vi "Read_Instr.vi"(8 "error in (no error)":errorcluster caption="entrée d'erreur (pas d'erreur)", 11 "Class Instrument Multimeter en entrée":refnum<class "Class Instrument LED_Analyser.lvclass">) -> (0 "error out":errorcluster caption="sortie d'erreur", 3 "Class Instrument Multimeter en sortie":refnum<class "Class Instrument LED_Analyser.lvclass">)   [LabVIEW 2020, in "Library Instrument & Equipement.lvlib" / "Library Instruments.lvlib" / "Class Instrument LED_Analyser.lvclass"]
uses:
  Class Instrument LED_Analyser.lvclass
  Class Instrument LED_Analyser.lvclass/Class Instrument LED_Analyser.ctl
  Instrument (Default)/Class Instrument (Default).lvclass
  LED Analyser/Class Led Analyser (Default)/Class LED Analyser (Default).lvclass
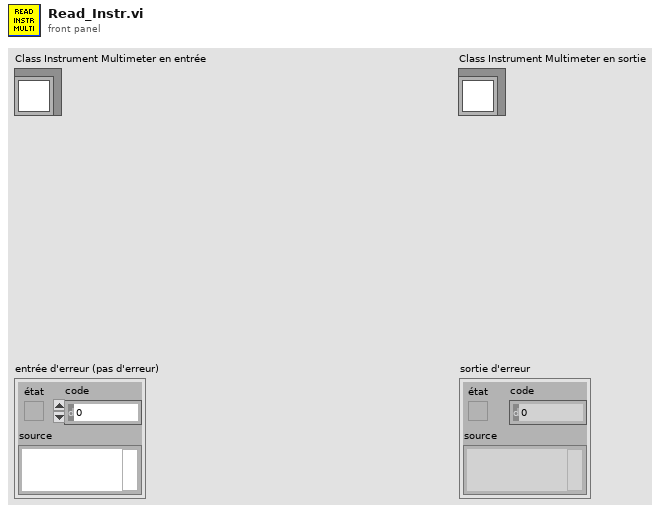
[diagram p1: front panel]
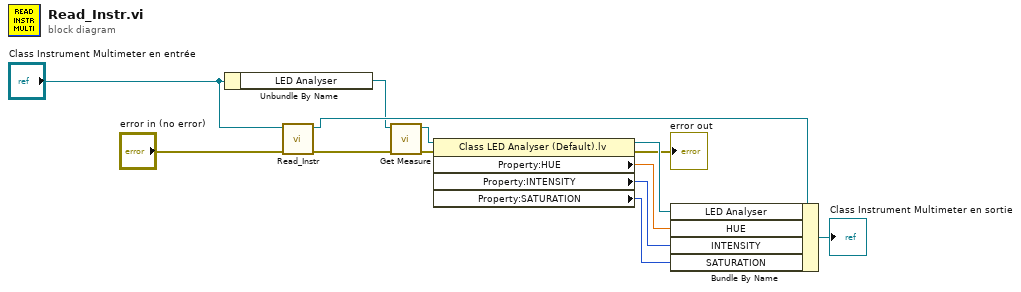
[diagram p0: block diagram]
diagram:
  n1 = Unbundle By Name("Class Instrument Multimeter en entrée") -> ("LED Analyser"=w2:refnum<class "Class LED Analyser (Default).lvclass">)
  n2 = call-parent "Read_Instr.vi"("error in (no error)"="error in (no error)", "Class Instrument (Default) en entrée"="Class Instrument Multimeter en entrée") -> ("error out"=w5:errorcluster, "Class Instrument (Default) en sortie"=w6:refnum<class "Class Instrument LED_Analyser.lvclass">)  [unwired: 8 in]
  n3 = call-dynamic "Get Measure.vi"("error in (no error)"=w5, "Class LED Analyser in"=w2) -> ("error out"=w4:errorcluster, "Class LED Analyser Out"=w3:refnum<class "Class LED Analyser (Default).lvclass">)  [unwired: 8 in]
  n4 = property class="Class LED Analyser (Default).lv"(reference=w3, error in=w4) -> (reference out=w10:refnum<class "Class LED Analyser (Default).lvclass">, error out=→"error out":errorcluster, "Property:HUE"=w9:dbl, "Property:INTENSITY"=w8:u32, "Property:SATURATION"=w1:u32)
  n5 = Bundle By Name(cluster=w6, "LED Analyser"=w10, "HUE"=w9, "INTENSITY"=w8, "SATURATION"=w1) -> (→"Class Instrument Multimeter en sortie":refnum<class "Class Instrument LED_Analyser.lvclass">)
